vi "Cmd To Turn Off Modulation.vi"(11 "Channel (1: 1)":i32(ring)=1 items=["1"=1, "2"=2]) -> (3 "Cmd String":string)   [LabVIEW 2019, in "Agilent 3352X Series.lvlib"]
doc: "Returns the cmd string of turning off all the modulation."
uses:
  <instrlib>/Agilent 3352X Series/Agilent 3352X Series.lvlib
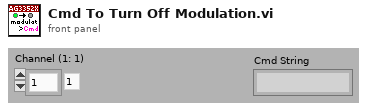
[diagram p1: front panel]
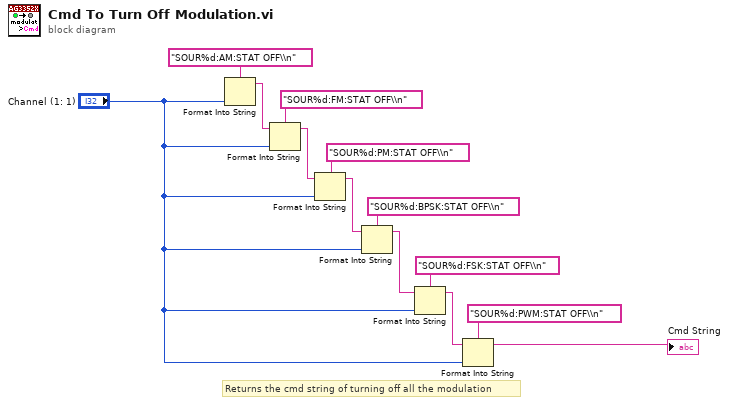
[diagram p0: block diagram]
diagram:
  # "Returns the cmd string of turning off all the modulation"
  n1 = Format Into String(format string="SOUR%d:AM:STAT OFF\\n", "Channel (1: 1)") -> (resulting string=w10:string)  [unwired: 2 in, 1 out]
  n2 = Format Into String(format string="SOUR%d:FM:STAT OFF\\n", initial string=w10, "Channel (1: 1)") -> (resulting string=w9:string)  [unwired: 1 in, 1 out]
  n3 = Format Into String(format string="SOUR%d:PM:STAT OFF\\n", initial string=w9, "Channel (1: 1)") -> (resulting string=w7:string)  [unwired: 1 in, 1 out]
  n4 = Format Into String(format string="SOUR%d:BPSK:STAT OFF\\n", initial string=w7, "Channel (1: 1)") -> (resulting string=w5:string)  [unwired: 1 in, 1 out]
  n5 = Format Into String(format string="SOUR%d:FSK:STAT OFF\\n", initial string=w5, "Channel (1: 1)") -> (resulting string=w3:string)  [unwired: 1 in, 1 out]
  n6 = Format Into String(format string="SOUR%d:PWM:STAT OFF\\n", initial string=w3, "Channel (1: 1)") -> (resulting string=→"Cmd String":string)  [unwired: 1 in, 1 out]
